vi "Simulator VNA Measure.vi"(8 "error in (no error)":errorcluster, 10 "SP Stimulus":T5={"Use Instrument Settings"=FALSE, "Blank Frequencies"=FALSE, "Sweep Type"=enum."Linear", "Sweep"={"Fstart"=500.0, "Fstop"=1500.0, "Units"=enum."MHz", "Points"=201}, "Power (dBm)"=999.0, "IFBW (Hz)"=-1.0, "Sweep Time (s)"=-1.0, "Calibration"={"State"=FALSE, "String"=""}} {"Sweep Time (s)" format="%.3g"}, 11 "Parameters to Measure":T1[](array[typedef]) {"Channel" min=1 max=99 step=1; "Parameter"."Stimulus Port" min=1 step=1; "Parameter"."Response Port" min=1 step=1}) -> (0 "error out":errorcluster, 2 "S Parameters":cluster{"f0":dbl, "df":dbl, cdb[][]}, 3 "Parameters to Measure":T1[](array[typedef]) {"Channel" min=1 max=99 step=1; "Parameter"."Stimulus Port" min=1 step=1; "Parameter"."Response Port" min=1 step=1})   [LabVIEW 2011]
uses:
  tests/S Parameter/TypeDefs/SP Stimulus Parameters.ctl
  tests/S Parameter/TypeDefs/SP Frequency Units.ctl
  tests/S Parameter/TypeDefs/SP Calibration State.ctl
  tests/S Parameter/TypeDefs/SP Parameter to Measure.ctl
  tests/S Parameter/TypeDefs/SP Parameter.ctl
  tests/S Parameter/TypeDefs/SP Measurement Format.ctl
panel:
  out "Plot S12":cluster{"f0":dbl, "df":dbl, dbl[][]}(graph)
  out "Plot S22":cluster{"Fstart, MHz":dbl, dbl, dbl[][]}(graph)
  out "Plot S21":cluster{"f0":dbl, "df":dbl, dbl[][]}(graph)
  out "Plot S11":cluster{"Fstart, MHz":dbl, dbl, dbl[][]}(graph)
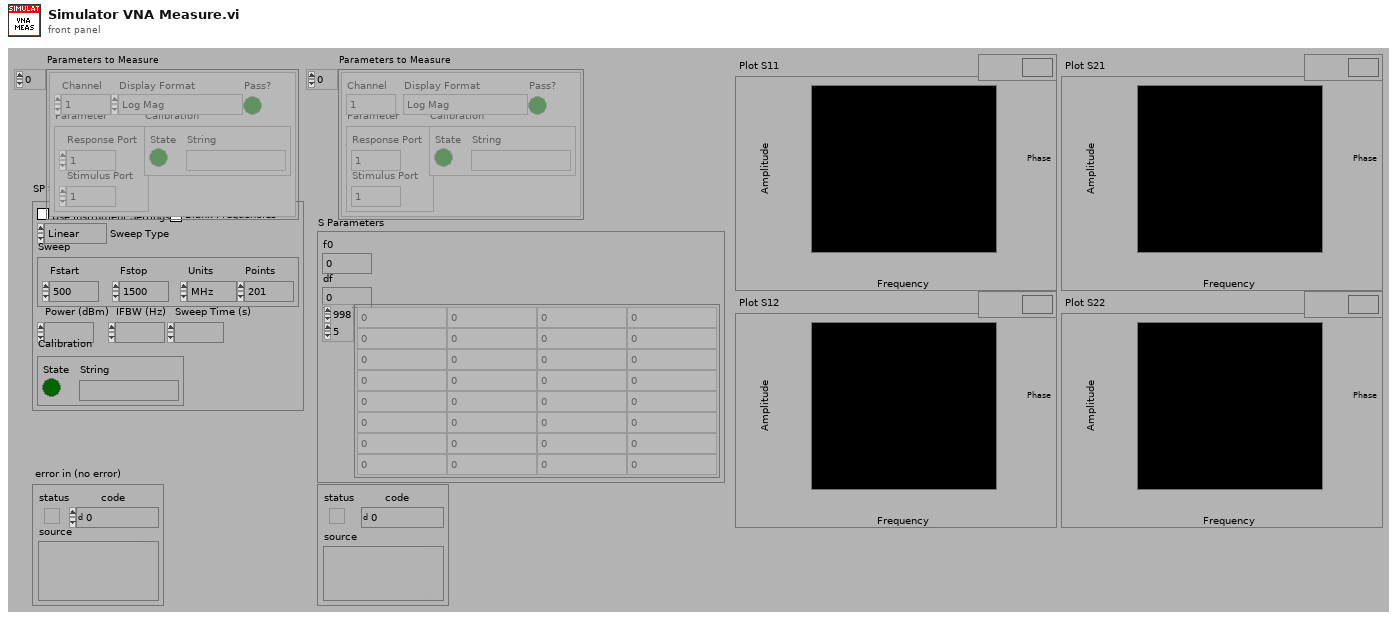
[diagram p1: front panel]
types:
  T1 = typedef "SP Parameter to Measure.ctl" = cluster{"Channel":i8, "Parameter":T2, "Calibration":T3, "Display Format":T4, "Pass?":bool}
  T2 = typedef "SP Parameter.ctl" = cluster{"Stimulus Port":i8, "Response Port":i8}
  T3 = typedef "SP Calibration State.ctl" = cluster{"State":bool, "String":string}
  T4 = typedef "SP Measurement Format.ctl" = enum32{"Log Mag", "Phase", "Delay", "Smith (R+jX)", "Polar (Re/Im)", "Linear Mag", "SWR", "Real", "Imaginary", "Smith (Lin/Phase)", "Smith (Log/Phase)", "Smith (Real/Imag)", "Smith (G+jB)", "Polar (Lin/Phase)", "Polar (Log/Phase)", "Expanded Phase", "Positive Phase", "Inverted Smith", "Unwrapped Phase", "Power Out", "Power In", "Linear Mag/Phase", "Log Mag/Phase", "Real/Imaginary"}
  T5 = typedef "SP Stimulus Parameters.ctl" = cluster{"Use Instrument Settings":bool, "Blank Frequencies":bool, "Sweep Type":enum32{"Linear", "Logarithmic", "List", "Power", "CW"}, "Sweep":cluster{"Fstart":dbl, "Fstop":dbl, "Units":T6, "Points":i32}, "Power (dBm)":dbl, "IFBW (Hz)":dbl, "Sweep Time (s)":dbl, "Calibration":T3}
  T6 = typedef "SP Frequency Units.ctl" = enum16{"Hz", "kHz", "MHz", "GHz", "Points"}
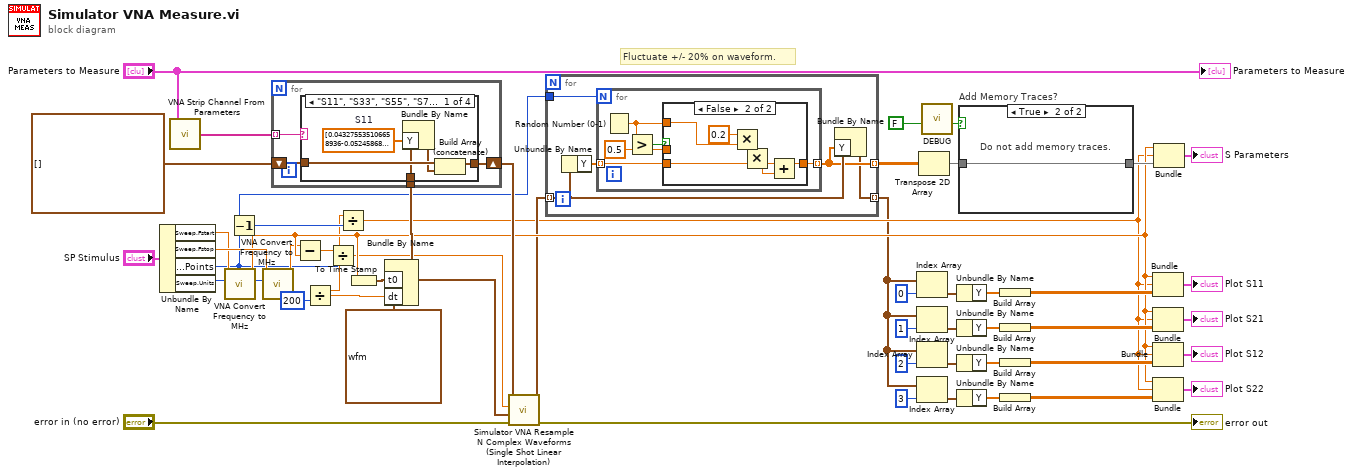
[diagram p0: block diagram]
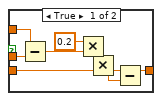
[diagram p2: hidden frame]
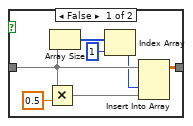
[diagram p3: hidden frame]
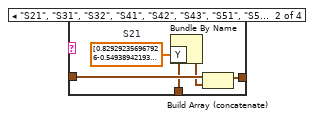
[diagram p4: hidden frame]
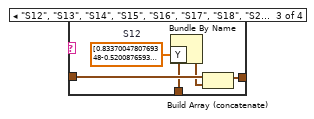
[diagram p5: hidden frame]
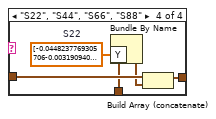
[diagram p6: hidden frame]
diagram:
  # "Fluctuate +/- 20% on waveform."
  n1 = Unbundle By Name("SP Stimulus") -> ("Sweep.Fstart"=w12:dbl, "Sweep.Fstop"=w13:dbl, "Sweep.Points"=w1:i32, "Sweep.Units"=w9:T6)
  n2 = call "VNA Strip Channel From Parameters.vi"("Parameters to Measure"="Parameters to Measure") -> ("Parameters to Measure"=w48:string[])  [unwired: 4 out]
  n3 = call "VNA Convert Frequency to MHz.vi"("Units"=w9, "Frequency"=w12) -> ("Converted Frequency"=w11:dbl)  [unwired: 9 out]
  n4 = Decrement(x=w1) -> (x-1=w6:i32)
  n5 = call "VNA Convert Frequency to MHz.vi"("Units"=w9, "Frequency"=w13) -> ("Converted Frequency"=w10:dbl)  [unwired: 9 out]
  n6 = Subtract(x=w10, y=w11) -> (x-y=w5:dbl)
  n7 = Divide(x=w5, y=200 ("Points")) -> (x/y=w28:dbl)
  n8 = Divide(x=w5, y=w1) -> (x/y=w4:dbl)
  n9 = Divide(x=w5, y=w6) -> (x/y=w3:dbl)
  n10 = To Time Stamp(1:w11) -> (0:w27:timestamp)
  n11 = Bundle By Name(cluster=waveform(cdb) {"t0"=timestamp(0 s since 1904-01-01), "dt"=1.0, "Y"=[]} ("output waveform"), "t0"=w27, "dt"=w28) -> (w32:waveform(cdb))
  n12 = for {
    tunnel: w48 -> [w52] mode=indexing
    shift-right: [w53] -> w30
    shift-left: waveform(cdb)[] [] -> [w54]
    tunnel: w32 -> [w51]
    n13 = case shown="\"S11\", \"S33\", \"S55\", \"S77\", Default" w52 {
      tunnel: w54 -> [w59 w64 w69 w74]
      tunnel: [w58 w63 w68 w73] -> w53
      tunnel: w51 -> [w57 w62 w67 w72]
      frame "S11", "S33", "S55", "S77", Default {
        w56 = cdb[] [0.043275535106658936-0.05245868116617203i, 0.039342574775218964-0.05071653425693512i, 0.03575783222913742-0.04884551092982292i, 0.032080549746751785-0.04723075032234192i, 0.028698638081550598-0.045584786683321i, 0.025614049285650253-0.04328160732984543i, 0.02282632142305374-0.04142192751169205i, 0.020214837044477463-0.03897164389491081i, 0.018059048801660538-0.03719286620616913i, 0.015805359929800034-0.035114482045173645i, 0.014122397638857365-0.03333842754364014i, 0.012394579127430916-0.03198646754026413i, 0.010067702271044254-0.030141184106469154i, 0.008520152419805527-0.028375955298542976i, 0.007258761674165726-0.026841409504413605i, 0.005761267151683569-0.024879861623048782i, 0.00486418791115284-0.02313334308564663i, 0.0033858772367239-0.021516310051083565i, 0.002761210547760129-0.02036347985267639i, 0.0017304427456110716-0.018724005669355392i, 0.0012977475998923182-0.01720506325364113i, 0.0004616621881723404-0.015729913488030434i, -1.719485044304747e-05-0.014889072626829147i, -0.00042151467641815543-0.013263088651001453i, -0.0007105278200469911-0.011781997047364712i, -0.0012685193214565516-0.010829365812242031i, -0.0019677081145346165-0.009644937701523304i, -0.0026351099368184805-0.008749132975935936i, -0.0033787309657782316-0.007702108472585678i, -0.004169062245637178-0.006119612138718367i, -0.004505419172346592-0.004736927337944508i, -0.00413671275600791-0.0033264632802456617i, -0.0035033696331083775-0.002244185423478484i, -0.003271963680163026-0.0012471904046833515i, -0.003496718592941761-0.0013772252714261413i, -0.003873205743730068-0.0006305294227786362i, -0.003999741747975349+0.0006247073761187494i, -0.003930048085749149+0.0012243101373314857i, -0.003324817167595029+0.0020987309981137514i, -0.0031607337296009064+0.002581748180091381i, -0.0030308200512081385+0.0031974148005247116i, -0.0034498628228902817+0.0035445920657366514i, -0.003611180931329727+0.004769172053784132i, -0.0037343313451856375+0.006552339531481266i, -0.002879899460822344+0.007479402236640453i, -0.002135245129466057+0.008235395886003971i, -0.001469879411160946+0.008991935290396214i, -0.0009730787132866681+0.008853754960000515i, -0.0011905874125659466+0.009129215963184834i, -0.0010869997786357999+0.009620561264455318i, -0.0010538013884797692+0.010348744690418243i, -0.000801632646471262+0.010489259846508503i, -0.0003287283470854163+0.01074668113142252i, -0.00020402256632223725+0.011179725639522076i, -0.0002642142935656011+0.011779340915381908i, -0.00013643794227391481+0.01236088015139103i, 0.0005306923994794488+0.012881748378276825i, 0.0014401909429579973+0.0132743613794446i, 0.002155429683625698+0.013405581936240196i, 0.0026408841367810965+0.013723139651119709i, 0.002987817395478487+0.013528610579669476i, 0.0032288457732647657+0.01342017948627472i, 0.00361762847751379+0.01351323164999485i, 0.0037104820366948843+0.013639203272759914i, 0.004260951653122902+0.013640777207911015i, 0.0044131227768957615+0.014399070292711258i, 0.005049579311162233+0.014325296506285667i, 0.0053521208465099335+0.014584374614059925i, 0.006191197317093611+0.014676371589303017i, 0.00685926852747798+0.014775711111724377i, 0.007911991328001022+0.014558723196387291i, 0.008351437747478485+0.014308781363070011i, 0.008801144547760487+0.013984980061650276i, 0.008953887969255447+0.01394110918045044i, 0.009607013314962387+0.013872258365154266i, 0.010086072608828545+0.014237764291465282i, 0.010762657038867474+0.014534384943544865i, 0.011188128031790257+0.014584838412702084i, 0.011861111968755722+0.01460554450750351i, 0.012636076658964157+0.014309742487967014i, 0.01329171285033226+0.014256738126277924i, 0.01419072039425373+0.014315866865217686i, 0.014360726810991764+0.01412278600037098i, 0.014936965890228748+0.013785612769424915i, 0.014871757477521896+0.013374490663409233i, 0.015183527953922749+0.013054748997092247i, 0.015605935826897621+0.012982526794075966i, 0.015983808785676956+0.012641431763768196i, 0.01635676436126232+0.012408261187374592i, 0.0168494563549757+0.01209751982241869i, 0.01760626956820488+0.011532459408044815i, 0.018216129392385483+0.010751352645456791i, 0.018974874168634415+0.009943358600139618i, 0.019734209403395653+0.008982783183455467i, 0.01982462778687477+0.008071470074355602i, 0.02016322687268257+0.007421128451824188i, 0.02022622525691986+0.006713556125760078i, 0.020693926140666008+0.006053129676729441i, 0.020658815279603004+0.005938771180808544i, 0.021412502974271774+0.005330209154635668i, 0.021840233355760574+0.004900768864899874i, 0.02223920449614525+0.004284977447241545i, 0.022984003648161888+0.0033651182893663645i, 0.023274244740605354+0.002730223350226879i, 0.0235948096960783+0.0015676334733143449i, 0.023692430928349495+0.0005109593039378524i, 0.023691050708293915-0.0005398404318839312i, 0.023721178993582726-0.0019432937260717154i, 0.023409923538565636-0.0026937827933579683i, 0.02332262136042118-0.0033581224270164967i, 0.0232867244631052-0.004046980291604996i, 0.023343225941061974-0.004525003954768181i, 0.02331232838332653-0.005694722291082144i, 0.023639868944883347-0.006385371554642916i, 0.023666899651288986-0.007270871661603451i, 0.023931000381708145-0.008271224796772003i, 0.024006182327866554-0.009296927601099014i, 0.024024013429880142-0.010424446314573288i, 0.02399740368127823-0.011644992046058178i, 0.02352958731353283-0.01281037274748087i, 0.02293366566300392-0.0136734489351511i, 0.022277450188994408-0.015110677108168602i, 0.02165168710052967-0.015935854986310005i, 0.021030226722359657-0.01672895811498165i, 0.020597459748387337-0.01770201325416565i, 0.019762272015213966-0.01837054267525673i, 0.01981099136173725-0.01910082809627056i, 0.0190260112285614-0.02045709453523159i, 0.01884141005575657-0.021298810839653015i, 0.018474403768777847-0.02227306179702282i, 0.018153464421629906-0.023544836789369583i, 0.017230894416570663-0.024686085060238838i, 0.01683255285024643-0.02567151002585888i, 0.015972070395946503-0.027068637311458588i, 0.014567862264811993-0.027528198435902596i, 0.013760950416326523-0.028633495792746544i, 0.012620450928807259-0.029594412073493004i, 0.010907035320997238-0.03021681122481823i, 0.009974002838134766-0.030786173418164253i, 0.00895930826663971-0.03156764805316925i, 0.007833925075829029-0.03187621384859085i, 0.007271322887390852-0.03240183740854263i, 0.006285695359110832-0.033501096069812775i, 0.005394641775637865-0.034671850502491i, 0.004059544298797846-0.035739753395318985i, 0.002686774358153343-0.036603860557079315i, 0.0017567717004567385-0.037068404257297516i, 0.0006243944517336786-0.03781891241669655i, -0.0004936228506267071-0.03891896829009056i, -0.0028370742220431566-0.03973366692662239i, -0.005315746646374464-0.03967787325382233i, -0.0071689714677631855-0.03857695311307907i, -0.007896475493907928-0.03817327320575714i, -0.008393912576138973-0.03789934515953064i, -0.009499276988208294-0.03860495984554291i, -0.010864137671887875-0.039575327187776566i, -0.013279550708830357-0.040249649435281754i, -0.015229152515530586-0.040115803480148315i, -0.016355840489268303-0.03987248241901398i, -0.01756197027862072-0.040174949914216995i, -0.018781857565045357-0.041554514318704605i, -0.021512817591428757-0.042375631630420685i, -0.025313854217529297-0.042042654007673264i, -0.027553554624319077-0.040576834231615067i, -0.028660070151090622-0.037809837609529495i, -0.028027910739183426-0.035897962749004364i, -0.02755579724907875-0.036189399659633636i, -0.028688842430710793-0.03706051781773567i, -0.03104601986706257-0.03752564266324043i, -0.03363754600286484-0.036627382040023804i, -0.03597893938422203-0.03453949838876724i, -0.03675049543380737-0.032771121710538864i, -0.03752102330327034-0.03258080780506134i, -0.03978640213608742-0.03393174707889557i, -0.042819179594516754-0.033820636570453644i, -0.047085169702768326-0.03167271614074707i, -0.049191735684871674-0.027427541092038155i, -0.04951959848403931-0.024153072386980057i, -0.04790704324841499-0.022657835856080055i, -0.04758603125810623-0.02298768423497677i, -0.04839025065302849-0.02431694231927395i, -0.05057644844055176-0.02427603304386139i, -0.0533347986638546-0.02293049544095993i, -0.05488186329603195-0.020498810335993767i, -0.05515661835670471-0.018127398565411568i, -0.05508638545870781-0.01620027795433998i, -0.055647045373916626-0.015622779726982117i, -0.05629001185297966-0.013566534966230392i, -0.05946866795420647-0.012328879907727242i, -0.06072845682501793-0.008508511818945408i, -0.06155878305435181-0.004364722408354282i, -0.0606592521071434-0.0013175384374335408i, -0.060178909450769424+0.0007016356103122234i, -0.05885367840528488+0.0017052150797098875i, -0.06058591604232788+0.0030290342401713133i, -0.06147431954741478+0.004005967173725367i, -0.06279278546571732+0.005614572670310736i, -0.06465675681829453+0.008378111757338047i, -0.06480240076780319+0.011182919144630432i, -0.06487281620502472+0.014382719062268734i, -0.06429072469472885+0.01689312979578972i]  # S11
        n14 = Bundle By Name(cluster=w57, "Y"=w56) -> (w55:waveform(cdb))
        n15 = Build Array (concatenate)(w59, w55) -> (w58:waveform(cdb)[])
      }
      frame "S21", "S31", "S32", "S41", "S42", "S43", "S51", "S52", "S53", "S54", "S61", "S62", "S63", "S64", "S65", "S71", "S72", "S73", "S74", "S75", "S76", "S81", "S82", "S83", "S84", "S85", "S86", "S87" {
        w60 = cdb[] [0.829292356967926-0.5493894219398499i, 0.814454197883606-0.5690862536430359i, 0.7981213331222534-0.5927940011024475i, 0.7870112657546997-0.6100444793701172i, 0.7711793184280396-0.6289911866188049i, 0.7556583285331726-0.6504056453704834i, 0.7388772964477539-0.6671569347381592i, 0.7228282690048218-0.6846721172332764i, 0.7071607112884521-0.7030295133590698i, 0.6912792325019836-0.7181567549705505i, 0.6753528118133545-0.7356259822845459i, 0.6560407876968384-0.7493025064468384i, 0.6371591091156006-0.7641898989677429i, 0.6180185079574585-0.7797850966453552i, 0.6032703518867493-0.7939913272857666i, 0.5853940844535828-0.8093052506446838i, 0.5672386288642883-0.8234372138977051i, 0.5465737581253052-0.8317574262619019i, 0.5287693738937378-0.8441898822784424i, 0.5108529925346375-0.8575894832611084i, 0.4929536283016205-0.8689723014831543i, 0.4726460576057434-0.8790130019187927i, 0.45388948917388916-0.8885069489479065i, 0.4329501986503601-0.8994144201278687i, 0.41499051451683044-0.9069346189498901i, 0.3953711688518524-0.9155407547950745i, 0.37639090418815613-0.9246777296066284i, 0.35440051555633545-0.9296605587005615i, 0.3362242579460144-0.9379180669784546i, 0.31509923934936523-0.946359395980835i, 0.29575711488723755-0.9532225728034973i, 0.2755361497402191-0.9575815796852112i, 0.2568615674972534-0.9623299241065979i, 0.23595577478408813-0.9689970016479492i, 0.21444492042064667-0.9749433994293213i, 0.19693320989608765-0.9783788323402405i, 0.17813338339328766-0.9837055206298828i, 0.15588150918483734-0.9873795509338379i, 0.13776037096977234-0.9871167540550232i, 0.11660043895244598-0.9899600148200989i, 0.09747599810361862-0.9890207648277283i, 0.07880620658397675-0.9961696267127991i, 0.05615612864494324-0.9974749684333801i, 0.0381329171359539-0.9965118169784546i, 0.016294067725539207-0.9968450665473938i, -0.003492713673040271-0.9984539151191711i, -0.021831337362527847-0.9984779953956604i, -0.0421501062810421-0.9960582256317139i, -0.061345260590314865-0.9936347007751465i, -0.08185604959726334-0.9966854453086853i, -0.09892823547124863-0.9929929971694946i, -0.12116867303848267-0.9893215894699097i, -0.1380733698606491-0.98619145154953i, -0.15851135551929474-0.9845050573348999i, -0.1788916140794754-0.9848970174789429i, -0.19643454253673553-0.9799931049346924i, -0.21329368650913239-0.9739719033241272i, -0.2337159663438797-0.969589114189148i, -0.25253576040267944-0.9657691717147827i, -0.270393967628479-0.9631704688072205i, -0.2902970314025879-0.9542956948280334i, -0.3075717091560364-0.9506268501281738i, -0.32540351152420044-0.9424934983253479i, -0.3427804410457611-0.9356661438941956i, -0.358801931142807-0.9293452501296997i, -0.3782116174697876-0.9225648641586304i, -0.3964827358722687-0.9151864647865295i, -0.4130129814147949-0.9065918922424316i, -0.42976996302604675-0.899314820766449i, -0.44708988070487976-0.891536295413971i, -0.4636856019496918-0.8827106356620789i, -0.48080843687057495-0.8736503720283508i, -0.4962398409843445-0.8642979264259338i, -0.5128710269927979-0.8545191884040833i, -0.5280305743217468-0.8468981981277466i, -0.5448092818260193-0.836822509765625i, -0.5582361817359924-0.8243995308876038i, -0.5728786587715149-0.8136676549911499i, -0.5888417363166809-0.806020200252533i, -0.6064391136169434-0.7927097678184509i, -0.6201893091201782-0.7820960879325867i, -0.6338473558425903-0.7690247893333435i, -0.6467384696006775-0.7588024735450745i, -0.6618889570236206-0.7466418147087097i, -0.676064670085907-0.7350124716758728i, -0.6866525411605835-0.720422089099884i, -0.7018538117408752-0.7068414092063904i, -0.7150512337684631-0.6946720480918884i, -0.728316068649292-0.6814172267913818i, -0.7392727136611938-0.6681946516036987i, -0.7518630027770996-0.6562276482582092i, -0.7645359635353088-0.6400392651557922i, -0.7738081812858582-0.6273608207702637i, -0.7883812189102173-0.6119368076324463i, -0.7997139096260071-0.5973165035247803i, -0.8098510503768921-0.5828021168708801i, -0.8207243084907532-0.5688458681106567i, -0.8297194838523865-0.5546996593475342i, -0.8402549028396606-0.5386097431182861i, -0.8492640852928162-0.5217608213424683i, -0.8584194183349609-0.5080013275146484i, -0.8675045371055603-0.4919714033603668i, -0.873566210269928-0.4768650531768799i, -0.8841186761856079-0.458417683839798i, -0.8934317827224731-0.4439525604248047i, -0.9010100960731506-0.4289016127586365i, -0.9081630110740662-0.41086092591285706i, -0.9165226817131042-0.39496952295303345i, -0.921902060508728-0.3788200616836548i, -0.929990291595459-0.3600974678993225i, -0.9349827766418457-0.34472861886024475i, -0.9424318671226501-0.3281252086162567i, -0.9459336996078491-0.3102380931377411i, -0.9520758390426636-0.29371288418769836i, -0.9587121605873108-0.2748992145061493i, -0.9634407162666321-0.2593393623828888i, -0.9670430421829224-0.24130849540233612i, -0.9712170362472534-0.22388198971748352i, -0.9760630130767822-0.20855499804019928i, -0.9790180325508118-0.1893032044172287i, -0.9799625277519226-0.17082269489765167i, -0.9845265746116638-0.1549006551504135i, -0.987425684928894-0.13725869357585907i, -0.989444375038147-0.11935828626155853i, -0.9929931163787842-0.10087912529706955i, -0.9935646057128906-0.08397430181503296i, -0.9969585537910461-0.06397698074579239i, -0.9946895837783813-0.046858273446559906i, -0.9962232708930969-0.030795134603977203i, -0.9964486360549927-0.010752464644610882i, -0.9962095022201538+0.006633169949054718i, -0.996056318283081+0.023876648396253586i, -0.9940896034240723+0.040969278663396835i, -0.9956469535827637+0.0587850958108902i, -0.9917272329330444+0.07762134075164795i, -0.9910922646522522+0.09390082210302353i, -0.9918628334999084+0.11216963082551956i, -0.986739456653595+0.1285705417394638i, -0.9865198731422424+0.14573192596435547i, -0.9832531809806824+0.1657622903585434i, -0.980251669883728+0.18302786350250244i, -0.9778366088867188+0.20167437195777893i, -0.972420334815979+0.2177964746952057i, -0.9679995179176331+0.2366965115070343i, -0.9628635048866272+0.25112852454185486i, -0.9585220813751221+0.2678850591182709i, -0.9528169631958008+0.2847737669944763i, -0.9470780491828918+0.301191508769989i, -0.9426121711730957+0.3168991208076477i, -0.9383622407913208+0.33460086584091187i, -0.9331514835357666+0.35213959217071533i, -0.9263299703598022+0.3680362403392792i, -0.9203755259513855+0.38593557476997375i, -0.913105309009552+0.40319201350212097i, -0.9034777283668518+0.4192873239517212i, -0.8951209187507629+0.43701618909835815i, -0.8883877992630005+0.4508943557739258i, -0.879611074924469+0.464642196893692i, -0.8694924712181091+0.48128756880760193i, -0.8617876768112183+0.49485471844673157i, -0.853515088558197+0.5074177384376526i, -0.8449181318283081+0.5218229293823242i, -0.8350080251693726+0.537224531173706i, -0.8312739729881287+0.5533552765846252i, -0.8206787109375+0.5724490880966187i, -0.8102623820304871+0.5874285697937012i, -0.7970291376113892+0.602837324142456i, -0.7831966876983643+0.6162238121032715i, -0.7730605602264404+0.630071222782135i, -0.7591240406036377+0.643388569355011i, -0.7464131116867065+0.6541889309883118i, -0.7364375591278076+0.6667038202285767i, -0.7251046299934387+0.6750170588493347i, -0.7161509394645691+0.6882807612419128i, -0.7067240476608276+0.7015341520309448i, -0.6938031315803528+0.713338315486908i, -0.6799384355545044+0.7273160815238953i, -0.6680499315261841+0.743193507194519i, -0.6545169353485107+0.7573610544204712i, -0.6385235786437988+0.7678831219673157i, -0.6245161294937134+0.7805160284042358i, -0.6076085567474365+0.7895139455795288i, -0.5907292366027832+0.7981275320053101i, -0.5797586441040039+0.807086169719696i, -0.5657033920288086+0.8169502019882202i, -0.5516921877861023+0.8245164752006531i, -0.5354703664779663+0.8333539962768555i, -0.523349404335022+0.8426549434661865i, -0.5107196569442749+0.8532902598381042i, -0.49576160311698914+0.8619523048400879i, -0.48084160685539246+0.8741511702537537i, -0.4637007713317871+0.8826679587364197i, -0.44816768169403076+0.8924193978309631i, -0.42999717593193054+0.9009377956390381i, -0.413239449262619+0.9052014946937561i, -0.3964954614639282+0.915328323841095i, -0.37846991419792175+0.9190049171447754i, -0.36190730333328247+0.927216112613678i, -0.3453793525695801+0.9306579232215881i, -0.32939761877059937+0.9367430210113525i, -0.31479111313819885+0.9424533843994141i]  # S21
        n16 = Bundle By Name(cluster=w62, "Y"=w60) -> (w61:waveform(cdb))
        n17 = Build Array (concatenate)(w64, w61) -> (w63:waveform(cdb)[])
      }
      frame "S12", "S13", "S14", "S15", "S16", "S17", "S18", "S23", "S24", "S25", "S26", "S27", "S28", "S34", "S35", "S36", "S37", "S38", "S45", "S46", "S47", "S48", "S56", "S57", "S58", "S67", "S68", "S78" {
        w65 = cdb[] [0.8337004780769348-0.5200876593589783i, 0.8181808590888977-0.5427855253219604i, 0.8031412959098816-0.5626685619354248i, 0.7909902334213257-0.5810166597366333i, 0.7788154482841492-0.6014497876167297i, 0.7681070566177368-0.6200025081634521i, 0.7551140785217285-0.643835723400116i, 0.7417704463005066-0.665276288986206i, 0.7248368859291077-0.6899394989013672i, 0.7070673704147339-0.713118314743042i, 0.6861556768417358-0.7328734993934631i, 0.6654462218284607-0.7541669607162476i, 0.637874960899353-0.7698982954025269i, 0.6171132922172546-0.7821155190467834i, 0.5911676287651062-0.7934721112251282i, 0.5713427066802979-0.7998170852661133i, 0.5516795516014099-0.8089763522148132i, 0.5347855091094971-0.8159884810447693i, 0.5204638242721558-0.822722852230072i, 0.5077767372131348-0.8331564664840698i, 0.4974057078361511-0.8450263142585754i, 0.4838629364967346-0.8576574921607971i, 0.46762534976005554-0.8765296339988708i, 0.4514274597167969-0.8934423327445984i, 0.4292939007282257-0.911008358001709i, 0.40243837237358093-0.9277858138084412i, 0.37349605560302734-0.9436126947402954i, 0.34189796447753906-0.9478856921195984i, 0.3098517060279846-0.953731894493103i, 0.2839166820049286-0.9518901109695435i, 0.2591840326786041-0.944251537322998i, 0.24050498008728027-0.9412912130355835i, 0.2294185906648636-0.9329850077629089i, 0.2192041575908661-0.9318305253982544i, 0.21159739792346954-0.9351982474327087i, 0.2037205696105957-0.9447835683822632i, 0.19587396085262299-0.9597285389900208i, 0.17845891416072845-0.9758542776107788i, 0.15374864637851715-0.9931191205978394i, 0.12296313047409058-1.009406566619873i, 0.08836781978607178-1.017944097518921i, 0.05404189974069595-1.0180165767669678i, 0.021986862644553185-1.009894847869873i, -0.00695606367662549-0.9979780316352844i, -0.028587350621819496-0.9817920923233032i, -0.04182153567671776-0.9717605710029602i, -0.05166104435920715-0.960070013999939i, -0.05838768184185028-0.956571102142334i, -0.06793583929538727-0.9588659405708313i, -0.07563966512680054-0.9689611792564392i, -0.09253257513046265-0.9764518737792969i, -0.11477933824062347-0.9877933263778687i, -0.13989581167697906-0.9933593273162842i, -0.17279675602912903-0.9930545091629028i, -0.20106659829616547-0.9880343079566956i, -0.22970663011074066-0.9796702265739441i, -0.25439924001693726-0.9658750891685486i, -0.2693353295326233-0.948691725730896i, -0.2889915406703949-0.9355658888816833i, -0.29486438632011414-0.9278984069824219i, -0.3078099489212036-0.9229747653007507i, -0.32018768787384033-0.9180485606193542i, -0.33861541748046875-0.9151418209075928i, -0.3564850091934204-0.9145493507385254i, -0.3752939999103546-0.9108543395996094i, -0.3948507308959961-0.902382493019104i, -0.41648608446121216-0.893722414970398i, -0.43723639845848083-0.8821430802345276i, -0.452502578496933-0.870651125907898i, -0.46733251214027405-0.8577056527137756i, -0.48071280121803284-0.8466469645500183i, -0.49225661158561707-0.8390735983848572i, -0.506791889667511-0.8290392756462097i, -0.5197045803070068-0.821696400642395i, -0.5357764363288879-0.8147437572479248i, -0.5509658455848694-0.8076014518737793i, -0.5691072344779968-0.797868549823761i, -0.5897894501686096-0.7851457595825195i, -0.605778157711029-0.7720136046409607i, -0.6210479140281677-0.7577008605003357i, -0.6325191855430603-0.7427079677581787i, -0.6439656615257263-0.7280888557434082i, -0.6548815965652466-0.712942898273468i, -0.6662686467170715-0.7019703388214111i, -0.6743442416191101-0.690955400466919i, -0.6855710744857788-0.6820973753929138i, -0.7000376582145691-0.6692298054695129i, -0.7117102146148682-0.6608266830444336i, -0.7253685593605042-0.6484005451202393i, -0.7386612296104431-0.6352925300598145i, -0.7532441020011902-0.6215614676475525i, -0.765815794467926-0.6052665114402771i, -0.7768866419792175-0.5882886052131653i, -0.7853107452392578-0.5689247846603394i, -0.7932745218276978-0.5519700050354004i, -0.800614058971405-0.5396230220794678i, -0.8092449903488159-0.5247517228126526i, -0.8147201538085938-0.5116841197013855i, -0.8231639862060547-0.4987384080886841i, -0.830460250377655-0.48304519057273865i, -0.8419719338417053-0.47280433773994446i, -0.8522282838821411-0.45855116844177246i, -0.8624382019042969-0.44237688183784485i, -0.8695622086524963-0.4247681200504303i, -0.8771089315414429-0.4078901708126068i, -0.8840516209602356-0.39066848158836365i, -0.888999342918396-0.372587114572525i, -0.891585111618042-0.35802125930786133i, -0.8962506055831909-0.34414008259773254i, -0.9008564949035645-0.33127647638320923i, -0.9058078527450562-0.317383348941803i, -0.913115382194519-0.30332472920417786i, -0.9204257130622864-0.288968563079834i, -0.9283400774002075-0.27373743057250977i, -0.935961902141571-0.25519245862960815i, -0.9418730735778809-0.2368680089712143i, -0.9456731081008911-0.2183118313550949i, -0.9482985734939575-0.19848909974098206i, -0.9491007924079895-0.18077704310417175i, -0.9507501721382141-0.16483846306800842i, -0.9520665407180786-0.14982055127620697i, -0.9530963897705078-0.1336503028869629i, -0.9568275213241577-0.12132811546325684i, -0.9600855112075806-0.10448877513408661i, -0.9627634882926941-0.0899454653263092i, -0.9671722650527954-0.07210934162139893i, -0.9694264531135559-0.05416249856352806i, -0.971646249294281-0.036692071706056595i, -0.972331702709198-0.01655270718038082i, -0.9724413156509399-0.0022197153884917498i, -0.9702968597412109+0.01574796810746193i, -0.9721423983573914+0.03205471113324165i, -0.9718196392059326+0.04803718253970146i, -0.9726036190986633+0.06537706404924393i, -0.9727047681808472+0.08238653093576431i, -0.9739677309989929+0.10253201425075531i, -0.9713402986526489+0.12144562602043152i, -0.9660041332244873+0.14094595611095428i, -0.960610032081604+0.1596621870994568i, -0.956613302230835+0.17383500933647156i, -0.9506188035011292+0.18698115646839142i, -0.948957622051239+0.202972412109375i, -0.9482381939888+0.21393731236457825i, -0.9498124122619629+0.22855278849601746i, -0.9518067240715027+0.24671871960163116i, -0.9508785605430603+0.2670695185661316i, -0.9477074146270752+0.2895950376987457i, -0.9427552819252014+0.3139152228832245i, -0.9327554702758789+0.3370639979839325i, -0.9165830612182617+0.35580992698669434i, -0.9024083018302917+0.3700178265571594i, -0.891497790813446+0.3783276081085205i, -0.8820448517799377+0.3841952383518219i, -0.8806410431861877+0.39001840353012085i, -0.8812286257743835+0.39776116609573364i, -0.88673335313797+0.4129319489002228i, -0.8888771533966064+0.4336598515510559i, -0.8925393223762512+0.45853614807128906i, -0.8883774876594543+0.4881307780742645i, -0.8752503395080566+0.5184275507926941i, -0.8541203737258911+0.5445005893707275i, -0.8287928104400635+0.5633280277252197i, -0.7984622716903687+0.5754674673080444i, -0.7784661054611206+0.5745667219161987i, -0.7642708420753479+0.5709152221679688i, -0.7597957253456116+0.5671483278274536i, -0.7634502649307251+0.5678656101226807i, -0.7701605558395386+0.5758752822875977i, -0.777458131313324+0.5932984352111816i, -0.7836854457855225+0.6184807419776917i, -0.781994640827179+0.651141881942749i, -0.7683941125869751+0.6870469450950623i, -0.7450302839279175+0.7181825637817383i, -0.7109066247940063+0.7427770495414734i, -0.6751865148544312+0.7549855709075928i, -0.6423426270484924+0.7535695433616638i, -0.6172760128974915+0.7444217801094055i, -0.6061503291130066+0.7326382398605347i, -0.6009782552719116+0.7257084846496582i, -0.6047084927558899+0.722892165184021i, -0.613054096698761+0.7282046675682068i, -0.6205593943595886+0.7458376288414001i, -0.6221399307250977+0.7666267156600952i, -0.618950366973877+0.8002158403396606i, -0.6042948365211487+0.8314599394798279i, -0.5778829455375671+0.862019419670105i, -0.5433223843574524+0.8841695189476013i, -0.509933352470398+0.8958801627159119i, -0.4719630777835846+0.8984365463256836i, -0.4437721371650696+0.8871181011199951i, -0.4217017590999603+0.877078652381897i, -0.4115893244743347+0.866625964641571i, -0.4102535843849182+0.8590211868286133i, -0.4117880165576935+0.856845498085022i, -0.4139910340309143+0.862561821937561i, -0.4183366298675537+0.8778890371322632i, -0.4167386591434479+0.8994209170341492i, -0.4066200256347656+0.926336407661438i, -0.38806724548339844+0.9557477831840515i, -0.3580075204372406+0.982031524181366i, -0.3183501064777374+1.0004563331604004i]  # S12
        n18 = Bundle By Name(cluster=w67, "Y"=w65) -> (w66:waveform(cdb))
        n19 = Build Array (concatenate)(w69, w66) -> (w68:waveform(cdb)[])
      }
      frame "S22", "S44", "S66", "S88" {
        w70 = cdb[] [-0.0448237769305706-0.0031909409444779158i, -0.04102639853954315-0.003578298492357135i, -0.03737544268369675-0.0037918221205472946i, -0.034089814871549606-0.004378031007945538i, -0.030959470197558403-0.004858761560171843i, -0.028162462636828423-0.005125708878040314i, -0.02541796676814556-0.006091923452913761i, -0.023308314383029938-0.006894167512655258i, -0.02091742493212223-0.007511247415095568i, -0.018918225541710854-0.008161223493516445i, -0.017081458121538162-0.008896378800272942i, -0.015482684597373009-0.009813006967306137i, -0.014000953175127506-0.010476639494299889i, -0.01254727877676487-0.011254988610744476i, -0.011165780946612358-0.012076066806912422i, -0.010345423594117165-0.012749994173645973i, -0.009379100054502487-0.013148177415132523i, -0.00840721745043993-0.013938951306045055i, -0.007564597763121128-0.014369625598192215i, -0.006762946490198374-0.014965459704399109i, -0.0059876772575080395-0.015762168914079666i, -0.005517164245247841-0.016370706260204315i, -0.004945616703480482-0.016755348071455956i, -0.004484861623495817-0.01741243526339531i, -0.004106960259377956-0.01802552491426468i, -0.0040862238965928555-0.018641890957951546i, -0.004174944944679737-0.01898816227912903i, -0.003841354977339506-0.01933005079627037i, -0.004038045182824135-0.019783206284046173i, -0.0041593159548938274-0.01978379301726818i, -0.0044232625514268875-0.019599732011556625i, -0.0041390941478312016-0.019732462242245674i, -0.004399512894451618-0.01977614127099514i, -0.004216721281409264-0.019617516547441483i, -0.004327621776610613-0.019545720890164375i, -0.004233787301927805-0.01981654390692711i, -0.004186590202152729-0.019801277667284012i, -0.004376720171421766-0.019878048449754715i, -0.004460547119379044-0.0196684617549181i, -0.004746682476252317-0.019741281867027283i, -0.005126139149069786-0.019498663023114204i, -0.00522314989939332-0.019358662888407707i, -0.005602819379419088-0.01900799199938774i, -0.005595334339886904-0.01860913261771202i, -0.005792031995952129-0.018228357657790184i, -0.005758288316428661-0.017683394253253937i, -0.005966282915323973-0.017409665510058403i, -0.005686081945896149-0.016997648403048515i, -0.005799978971481323-0.016679877415299416i, -0.005790566559880972-0.01634107530117035i, -0.006069929338991642-0.01604008674621582i, -0.006077638361603022-0.015667129307985306i, -0.006143453996628523-0.015240166336297989i, -0.006082667037844658-0.014732113108038902i, -0.006236350629478693-0.014161228202283382i, -0.006148894317448139-0.013658835552632809i, -0.006158811971545219-0.013270117342472076i, -0.005938847549259663-0.012807438150048256i, -0.005814449395984411-0.012504386715590954i, -0.005655704066157341-0.012021793983876705i, -0.005622300785034895-0.011536293663084507i, -0.005354489199817181-0.011305506341159344i, -0.005245627369731665-0.010691221803426743i, -0.005094286985695362-0.010289422236382961i, -0.005099698435515165-0.010104155167937279i, -0.0047679501585662365-0.009593877010047436i, -0.004622514359652996-0.009187191724777222i, -0.004251937381923199-0.00874422024935484i, -0.004076929297298193-0.008421937003731728i, -0.0038552219048142433-0.008173706941306591i, -0.0036175204440951347-0.007856392301619053i, -0.0032895402982831-0.007768594194203615i, -0.0030748452991247177-0.0075556025840342045i, -0.0027343553956598043-0.007163476198911667i, -0.0026735644787549973-0.007148217409849167i, -0.0024386083241552114-0.006915162783116102i, -0.0022648742888122797-0.006690399255603552i, -0.0021435734815895557-0.006528554484248161i, -0.0020642667077481747-0.006329646799713373i, -0.0019470123806968331-0.006132075563073158i, -0.0016891410341486335-0.005893159657716751i, -0.001467305002734065-0.005719352979212999i, -0.001399420783855021-0.005582865793257952i, -0.0010558502981439233-0.005473996512591839i, -0.0008833135943859816-0.005348376929759979i, -0.000758141977712512-0.0051859295926988125i, -0.00048745161620900035-0.005115710664540529i, -0.0003483314940240234-0.005013156216591597i, -0.00028839983860962093-0.004964848514646292i, -6.241415394470096e-05-0.004872789140790701i, 5.908060848014429e-05-0.004937014542520046i, 0.00019588899158407003-0.004831728525459766i, 0.00027953420067206025-0.004761506803333759i, 0.00035175096127204597-0.0047147455625236034i, 0.0003388347977306694-0.004716338124126196i, 0.00045757752377539873-0.0046366979368031025i, 0.0004954376490786672-0.004575367551296949i, 0.0004994297050870955-0.004473790526390076i, 0.0004787541402038187-0.004432526417076588i, 0.0004915528697893023-0.004394272342324257i, 0.0004942804225720465-0.004317898768931627i, 0.0004837051674257964-0.004215982276946306i, 0.0004830575198866427-0.004179366398602724i, 0.00048056108062155545-0.004071427974849939i, 0.0004647464957088232-0.003978381864726543i, 0.00045925183803774416-0.0039333864115178585i, 0.00039012142224237323-0.003850033041089773i, 0.00036192749394103885-0.0037637404166162014i, 0.0003474172262940556-0.0036384325940161943i, 0.0003007917548529804-0.0035327314399182796i, 0.0002585411712061614-0.003482129191979766i, 0.00020978024986106902-0.003346635727211833i, 9.311280882684514e-05-0.003205877495929599i, 3.437729537836276e-05-0.0030748227145522833i, -2.6182860892731696e-05-0.002911030314862728i, -9.559790487401187e-05-0.0027312692254781723i, -0.00012796329974662513-0.0025247561279684305i, -0.00016629937454126775-0.002360462211072445i, -0.00018859354895539582-0.002140144817531109i, -0.00016769948706496507-0.001985291950404644i, -0.00018103173351846635-0.001796266296878457i, -0.00018724691472016275-0.0015912147937342525i, -0.0001743300526868552-0.0014163899468258023i, -0.0001649048354011029-0.0012246443657204509i, -0.00015603502106387168-0.0010193532798439264i, -0.00013644371938426048-0.0008304196526296437i, -9.474530816078186e-05-0.0006120093166828156i, -5.9985057305311784e-05-0.0004058258782606572i, 8.870118108461611e-06-0.00020282028708606958i, 9.934559784596786e-05-2.5176070266752504e-05i, 0.00018127325165551156+0.00017337668396066874i, 0.0002790482831187546+0.00039199006278067827i, 0.00038650145870633423+0.0005803335225209594i, 0.000505543255712837+0.0007531963638029993i, 0.0006492372485809028+0.0009020287543535233i, 0.000811923120636493+0.0010725089814513922i, 0.0009885950712487102+0.0012399621773511171i, 0.001171267475001514+0.0013506157556548715i, 0.001365330652333796+0.0014470539754256606i, 0.0015696100890636444+0.0015234538586810231i, 0.0017706482904031873+0.0016147868009284139i, 0.0019801591988652945+0.001605349243618548i, 0.002092361217364669+0.0017002156237140298i, 0.0023044664412736893+0.0017075886717066169i, 0.0025349468924105167+0.0018162375781685114i, 0.002791930455714464+0.0018298979848623276i, 0.0030656736344099045+0.0017995476955547929i, 0.0033251012209802866+0.001740268780849874i, 0.0036497320979833603+0.0016436392907053232i, 0.003974618390202522+0.001494038151577115i, 0.004179029725492001+0.0013613739283755422i, 0.004448150750249624+0.0010927021503448486i, 0.004605614580214024+0.0007669926853850484i, 0.004715103656053543+0.0006820614798925817i, 0.004872438497841358+0.00044049054849892855i, 0.005027373321354389+0.0002099816920235753i, 0.005337926093488932-6.502228643512353e-05i, 0.005487888585776091-0.0003248402790632099i, 0.005758954677730799-0.0006304772687144578i, 0.005848472472280264-0.0011413918109610677i, 0.006054707802832127-0.0015616797609254718i, 0.006243602838367224-0.0021629813127219677i, 0.006152447313070297-0.0026789747644215822i, 0.006166351027786732-0.003175552934408188i, 0.006093923468142748-0.003791477996855974i, 0.005887094419449568-0.0044150399044156075i, 0.0057772016152739525-0.004852078855037689i, 0.005688414443284273-0.005288145504891872i, 0.005684699863195419-0.005775182042270899i, 0.005622982047498226-0.006423992104828358i, 0.005431497003883123-0.007224175147712231i, 0.005171825643628836-0.008032376877963543i, 0.004884790629148483-0.008776065893471241i, 0.004366884473711252-0.009406034834682941i, 0.003925090655684471-0.010146105661988258i, 0.003188987961038947-0.010610239580273628i, 0.0027057796251028776-0.011458871886134148i, 0.0021417015232145786-0.01188242994248867i, 0.0015629694098606706-0.01242772489786148i, 0.0010502667864784598-0.01295468583703041i, 0.0004264943127054721-0.013618174009025097i, -7.472128345398232e-05-0.014185905456542969i, -0.0008630462107248604-0.015164329670369625i, -0.001326490775682032-0.01585821807384491i, -0.002498344052582979-0.01688726618885994i, -0.003656521439552307-0.017657626420259476i, -0.005031170789152384-0.018387652933597565i, -0.006442666053771973-0.018519790843129158i, -0.007896801456809044-0.01881493255496025i, -0.009163213893771172-0.019276220351457596i, -0.010341767221689224-0.01936732605099678i, -0.011778250336647034-0.019201701506972313i, -0.012648561969399452-0.01944117620587349i, -0.013558346778154373-0.020153788849711418i, -0.014745736494660378-0.02035050466656685i, -0.016558662056922913-0.020911652594804764i, -0.017478901892900467-0.02102949284017086i, -0.019446969032287598-0.021553659811615944i, -0.0211798045784235-0.021757150068879128i, -0.023336362093687057-0.021934092044830322i, -0.025581542402505875-0.021997427567839622i]  # S22
        n20 = Bundle By Name(cluster=w72, "Y"=w70) -> (w71:waveform(cdb))
        n21 = Build Array (concatenate)(w74, w71) -> (w73:waveform(cdb)[])
      }
    }
  }
  n22 = call "Simulator VNA Resample N Complex Waveforms (Single Shot Linear Interpolation).vi"("error in (no error)"="error in (no error)", "t0"=w27, "dt"=w4, "waveforms in"=w30) -> ("error out"=→"error out":errorcluster, "resampled waveforms out"=w8:waveform(cdb)[])  [unwired: 1 in, 5 out]
  n23 = for {
    tunnel: w8 -> [w78] mode=indexing
    tunnel: [w77] -> w7 mode=indexing
    tunnel: [w76] -> w2 mode=indexing
    tunnel: w1 -> [w75]
    n24 = Unbundle By Name(w78) -> ("Y"=w79:cdb[])
    n25 = for {
      N: w75 -> [_]
      tunnel: w79 -> [w83] mode=indexing
      tunnel: [w80] -> w77 mode=indexing
      w81 = 0.5 ("y")
      n26 = Random Number (0-1)() -> (number: 0 to 1=w82:dbl)
      n27 = Greater?(x=w82, y=w81) -> (0:w84:bool)
      n28 = case shown="False" w84 {
        tunnel: w83 -> [w87 w96]
        tunnel: w82 -> [w92 w93]
        tunnel: w81 -> [w91 _]
        tunnel: [w85 w94] -> w80
        frame True {
          n29 = Subtract(x=w92, y=w91) -> (x-y=w90:dbl)
          n30 = Multiply(x=0.2, y=w90) -> (x*y=w88:dbl)
          n31 = Multiply(x=w88, y=w87) -> (x*y=w86:cdb)
          n32 = Subtract(x=w87, y=w86) -> (x-y=w85:cdb)
        }
        frame False {
          n33 = Multiply(x=0.2, y=w93) -> (x*y=w97:dbl)
          n34 = Multiply(x=w97, y=w96) -> (x*y=w95:cdb)
          n35 = Add(x=w96, y=w95) -> (x+y=w94:cdb)
        }
      }
    }
    n36 = Bundle By Name(cluster=w78, "Y"=w77) -> (w76:waveform(cdb))
  }
  n37 = Index Array(array=w2, index=0 ("disabled index (col)")) -> (element=w21:waveform(cdb))
  n38 = Index Array(array=w2, index=1 ("disabled index (col)")) -> (element=w20:waveform(cdb))
  n39 = Index Array(array=w2, index=2 ("disabled index (col)")) -> (element=w19:waveform(cdb))
  n40 = Index Array(array=w2, index=3 ("disabled index (col)")) -> (element=w22:waveform(cdb))
  n41 = Transpose 2D Array(2D array=w7) -> (transposed array=w14:cdb[][])
  n42 = call "DEBUG.vi"("Dev DEBUG? (f)"=FALSE) -> ("DEBUG?"=w44:bool)  [unwired: 1 in, 5 out]
  n43 = Unbundle By Name(w21) -> ("Y"=w18:cdb[])
  n44 = Unbundle By Name(w20) -> ("Y"=w17:cdb[])
  n45 = Unbundle By Name(w19) -> ("Y"=w16:cdb[])
  n46 = Unbundle By Name(w22) -> ("Y"=w15:cdb[])
  n47 = case "Add Memory Traces?" shown="True" w44 {
    tunnel: [w104 w106] -> w46
    tunnel: w14 -> [w103 w106]
    frame False {
      n48 = Multiply(x=w103, y=0.5) -> (x*y=w99:cdb[][])
      n49 = Array Size(array=w103) -> (size(s)=w102:i32[])
      n50 = Index Array(array=w102, index=1) -> (element=w100:i32)
      n51 = Insert Into Array(array=w103, index (col)=w100, new element=w99) -> (w104:cdb[][])  [unwired: 1 in]
    }
    frame True {
      # "Do not add memory traces."
    }
  }
  n52 = Build Array(w18) -> (w39:cdb[][])
  n53 = Build Array(w17) -> (w40:cdb[][])
  n54 = Build Array(w16) -> (w41:cdb[][])
  n55 = Build Array(w15) -> (w42:cdb[][])
  n56 = Bundle("Converted Frequency"=w11, w3, w39) -> (→"Plot S11":cluster{"Converted Frequency":dbl, dbl, cdb[][]})  [unwired: 1 out]
  n57 = Bundle("Converted Frequency"=w11, w3, w40) -> (→"Plot S21":cluster{"Converted Frequency":dbl, dbl, cdb[][]})  [unwired: 1 out]
  n58 = Bundle("Converted Frequency"=w11, w3, w41) -> (→"Plot S12":cluster{"Converted Frequency":dbl, dbl, cdb[][]})  [unwired: 1 out]
  n59 = Bundle("Converted Frequency"=w11, w3, w42) -> (→"Plot S22":cluster{"Converted Frequency":dbl, dbl, cdb[][]})  [unwired: 1 out]
  n60 = Bundle("Converted Frequency"=w11, w3, w46) -> (→"S Parameters":cluster{"Converted Frequency":dbl, dbl, cdb[][]})  [unwired: 1 out]
  "Parameters to Measure" <- "Parameters to Measure"
